vi "RestoreWin.vi"(8 "error in (no error)":errorcluster, 11 "Window Name":string) -> (0 "error out":errorcluster)   [LabVIEW 2020, in "WinAPI.lvlib"]
uses:
  WinAPI.lvlib
  C:/Users/dzoni/Documents/NJ/Playground/LV/WinAPI/DLL/WinAPI.dll
  DLL/WinAPI.dll
panel:
  out "MinimizeWindow":bool
  out "MaximizeWindow":bool
  out "SetWindowToForeground":i32
  out "ShowWindow":bool
  out "RestoreWindow":bool
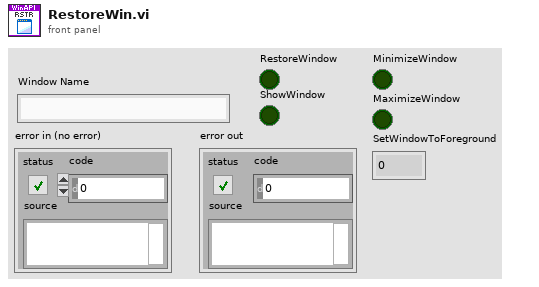
[diagram p1: front panel]
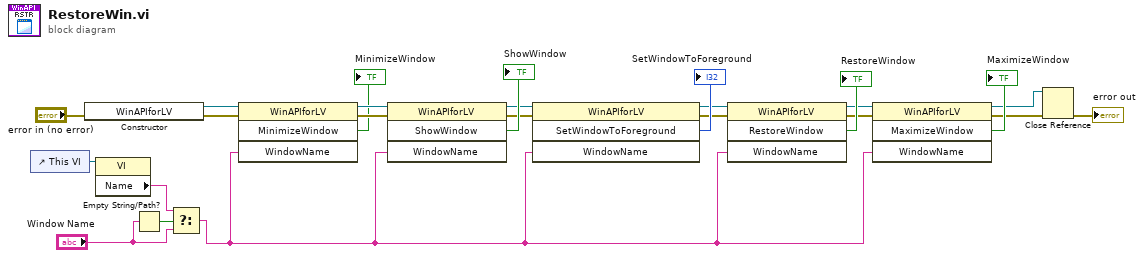
[diagram p0: block diagram]
diagram:
  n1 = control-ref of="This VI"() -> (w5:refnum<vi>)
  n2 = constructor class="WinAPIforLV"(error in="error in (no error)") -> (reference out=w13:refnum<k24>, error out=w14:errorcluster)  [unwired: 2 in, 1 out]
  n3 = property class="VI"(reference=w5) -> ("Name"=w4:string)  [unwired: 1 in, 2 out]
  n4 = Empty String/Path?(string/path="Window Name") -> (empty?=w3:bool)
  n5 = Select(t=w4, s=w3, f="Window Name") -> (s? t:f=w1:string)
  n6 = invoke class="WinAPIforLV" method="MinimizeWindow"(reference=w13, error in=w14, "WindowName"=w1) -> (reference out=w12:refnum<k24>, error out=w11:errorcluster, "MinimizeWindow"=→"MinimizeWindow":bool)  [unwired: 1 in, 1 out]
  n7 = invoke class="WinAPIforLV" method="ShowWindow"(reference=w12, error in=w11, "WindowName"=w1) -> (reference out=w18:refnum<k24>, error out=w17:errorcluster, "ShowWindow"=→"ShowWindow":bool)  [unwired: 1 in, 1 out]
  n8 = invoke class="WinAPIforLV" method="SetWindowToForeground"(reference=w18, error in=w17, "WindowName"=w1) -> (reference out=w15:refnum<k24>, error out=w16:errorcluster, "SetWindowToForeground"=→"SetWindowToForeground":i32)  [unwired: 1 in, 1 out]
  n9 = invoke class="WinAPIforLV" method="RestoreWindow"(reference=w15, error in=w16, "WindowName"=w1) -> (reference out=w9:refnum<k24>, error out=w8:errorcluster, "RestoreWindow"=→"RestoreWindow":bool)  [unwired: 1 in, 1 out]
  n10 = invoke class="WinAPIforLV" method="MaximizeWindow"(reference=w9, error in=w8, "WindowName"=w1) -> (reference out=w6:refnum<k24>, error out=w7:errorcluster, "MaximizeWindow"=→"MaximizeWindow":bool)  [unwired: 1 in, 1 out]
  n11 = Close Reference(reference=w6, error in (no error)=w7) -> (error out=→"error out":errorcluster)
